vi "MAVLink CRC v2.vi"   [LabVIEW 2014]
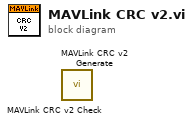
[diagram p0: block diagram]
diagram:
  n1 = call "MAVLink CRC v2 Check.vi"() -> ()  [unwired: 11 in, 1 out]
  n2 = call "MAVLink CRC v2 Generate.vi"() -> ()  [unwired: 11 in, 1 out]
